vi "Float Precision(lvlibp).vi"(8 "Enum":enum16{"Set", "Get"}(ring), 11 "Precision":string) -> (3 "Format String":string)   [LabVIEW 2017, in "API String Arguments Support.lvlib"]
uses:
  API String Arguments Support.lvlib
  Float Precision.vi
  <userlib>/_NEVSTOP/Communicable State Machine(CSM)/Communicable State Machine.lvlib
  <userlib>/_NEVSTOP/Communicable State Machine(CSM)/_Shared/CSM Shared.lvlib
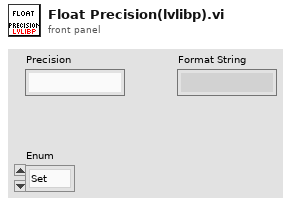
[diagram p1: front panel]
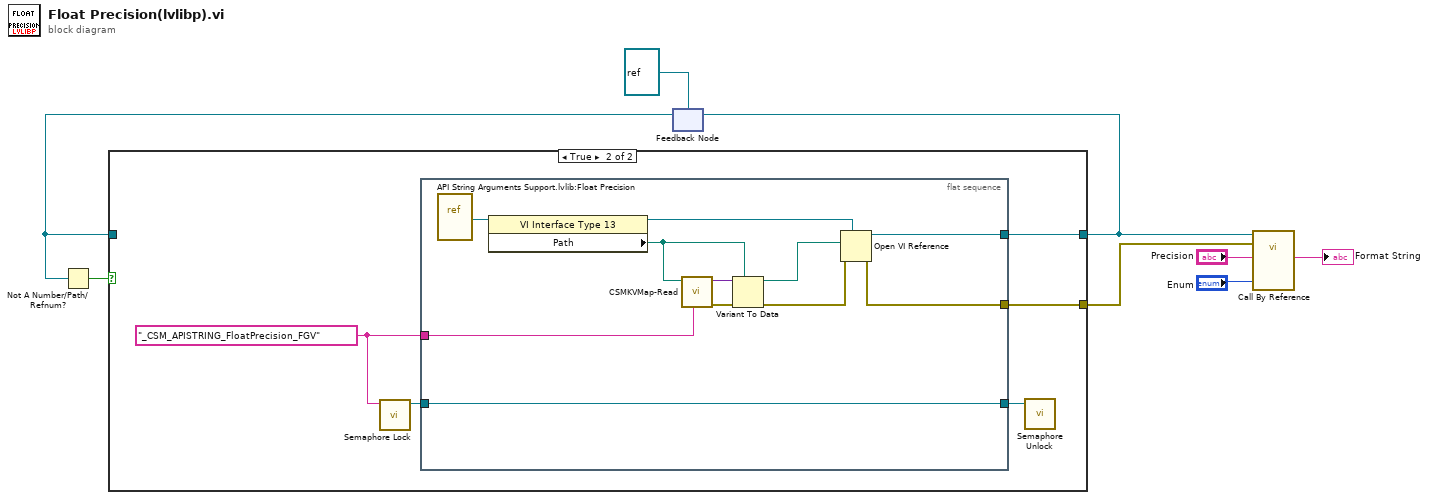
[diagram p0: block diagram]
diagram:
  n1 = feedback #1(refnum<vi> refnum) -> (w7:refnum<vi>)
  n2 = Not A Number/Path/Refnum?(number/path/refnum=w7) -> (NaN/Path/Refnum?=w8:bool)
  n3 = case shown="True" w8 {
    tunnel: [w9 w14] -> w5
    tunnel: w7 -> [w9 _]
    tunnel: [_ w13] -> w6
    frame False {
    }
    frame True {
      w10 = "_CSM_APISTRING_FloatPrecision_FGV" ("name")
      n4 = call <userlib>:"Semaphore Lock.vi"("name"=w10) -> ("semaphore"=w11:refnum<queue>)  [unwired: 10 in]
      n5 = flat-sequence {
        tunnel: [w17] -> w14
        tunnel: [w20] -> w13
        tunnel: w10 -> [w16]
        tunnel: [w15] -> w12
        tunnel: w11 -> [w15]
        frame #0 {
          n6 = vi-ref "API String Arguments Support.lvlib:Float Precision.vi"() -> (w25:refnum<vi>)
          n7 = property class="VI Interface Type 13"(reference=w25) -> (reference out=w18:refnum<vi>, "Path"=w22:path)  [unwired: 1 in, 1 out]
          n8 = call <userlib>:"CSMKVMap-Read.vi"("name"=w16, "default value (empty variant)"=w22) -> ("Error out"=w24:errorcluster, "value"=w23:variant)  [unwired: 6 in]
          n9 = Variant To Data(error in=w24, type=w22, Variant=w23) -> (data=w21:path, error out=w19:errorcluster)
          n10 = Open VI Reference(type specifier VI Refnum (for type only)=w18, vi path=w21, error in (no error)=w19) -> (vi reference=w17:refnum<vi>, error out=w20:errorcluster)  [unwired: 3 in]
        }
      }
      n11 = call <userlib>:"Semaphore Unlock.vi"("semaphore"=w12) -> ()  [unwired: 11 in]
    }
  }
  n12 = feedback-in #1(w5) -> ()
  n13 = call-by-ref "?"(reference=w5, error in=w6, "Enum"="Enum", "Precision"="Precision") -> ("Format String"=→"Format String":string)  [unwired: 9 in, 2 out]
